vi "MicroSlide-SendCmd.vi"(0 "VRN IN":refnum<visa-resource-name>="COM15", 2 "Commande":u16(ring) items=["Initialisation", "Mise dans le faisceau", "Retirer du faisceau"], 11 "Error IN":errorcluster) -> (4 "VRN OUT":refnum<visa-resource-name>="COM15", 8 "All cool !!!":bool, 15 "Error OUT":errorcluster)   [LabVIEW 2019]
panel:
  out "sent buffer":string
  out "read buffer":string
  out "Echo reçue":bool
  out "Commande envoyée":bool
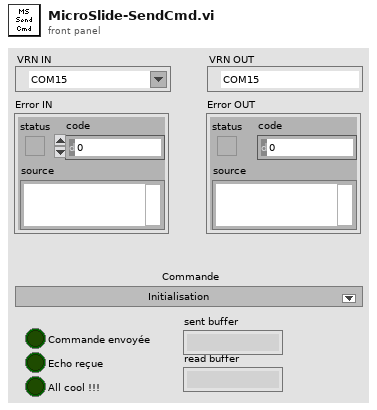
[diagram p1: front panel]
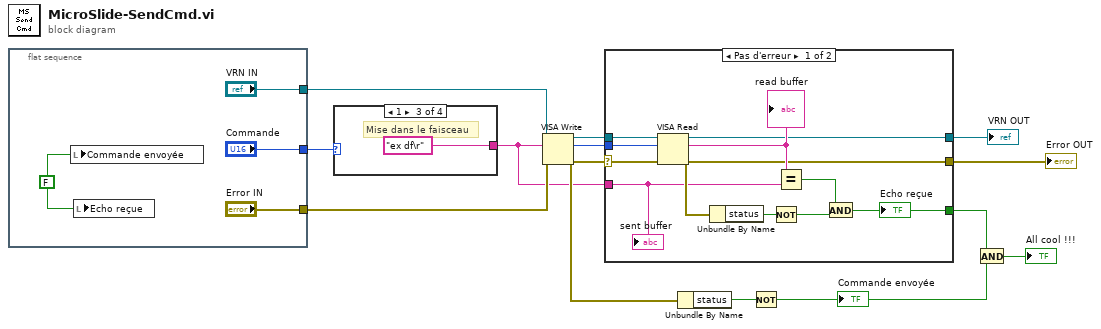
[diagram p0: block diagram]
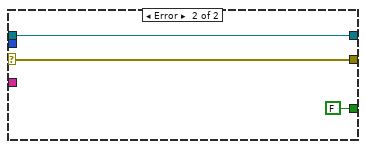
[diagram p2: hidden frame]
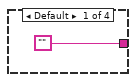
[diagram p3: hidden frame]
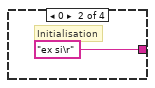
[diagram p4: hidden frame]
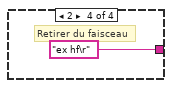
[diagram p5: hidden frame]
diagram:
  n1 = flat-sequence {
    tunnel: ["VRN IN"] -> w13
    tunnel: ["Error IN"] -> w12
    tunnel: ["Commande"] -> w11
    frame #0 {
      w16 = FALSE
      n2 = local write "Commande envoyée"(w16) -> ()
      n3 = local write "Echo reçue"(w16) -> ()
    }
  }
  n4 = case shown="1" w11 {
    tunnel: ["" "ex si\r" "ex df\r" "ex hf\r"] -> w6
    frame Default {
    }
    frame 0 {
      # "Initialisation"
    }
    frame 1 {
      # "Mise dans le faisceau"
    }
    frame 2 {
      # "Retirer du faisceau"
    }
  }
  n5 = VISA Write(VISA resource name=w13, write buffer=w6, error in (no error)=w12) -> (VISA resource name out=w7:refnum<visa-resource-name>, return count=w9:u32, error out=w8:errorcluster)
  n6 = case shown="Pas d'erreur" w8 {
    selector: w8 -> [w31 w34]
    tunnel: w9 -> [w32 _]
    tunnel: w7 -> [w30 w35]
    tunnel: w6 -> [w22 _]
    tunnel: [w25 w35] -> w4
    tunnel: [w24 w34] -> w5
    tunnel: [w23 FALSE] -> w2
    frame No Error {
      n7 = VISA Read(VISA resource name=w30, byte count=w32, error in (no error)=w31) -> (VISA resource name out=w25:refnum<visa-resource-name>, read buffer=w27:string, error out=w24:errorcluster)  [unwired: 1 out]
      "read buffer" <- w27
      n8 = Unbundle By Name(w24) -> ("status"=w29:bool)
      n9 = Not(x=w29) -> (.not. x?=w28:bool)
      n10 = Equal?(x=w27, y=w22) -> (x = y?=w26:bool)
      n11 = And(x=w26, y=w28) -> (x .and. y?=w23:bool)
      "Echo reçue" <- w23
      "sent buffer" <- w22
    }
    frame Error {
    }
  }
  "VRN OUT" <- w4
  "Error OUT" <- w5
  n12 = Unbundle By Name(w8) -> ("status"=w10:bool)
  n13 = Not(x=w10) -> (.not. x?=w3:bool)
  "Commande envoyée" <- w3
  n14 = And(x=w2, y=w3) -> (x .and. y?=→"All cool !!!":bool)
